vi "9217_UI.vi"(8 "error in (no error)":errorcluster, 11 "Node Ptr":T3 format="%.0x") -> (0 "error out":errorcluster)   [LabVIEW 2019, in "Modules.lvlib" / "9217.lvclass"]
uses:
  9217.lvclass
  <vilib>/NI VeriStand/Custom Device API/Custom Device Item Ref.ctl
  RSI Module/SubPanel Command.ctl
  _nicrio_cRIO-9217_SubPan_ConversionTime.ctl
  C:/Users/nitest/Desktop/Git 2019/niveristand-scan-engine-module-libraries/Source/RSI Module/RSI Module.lvclass
  9217.lvclass/9217.ctl
  RSI Module/RSI Module.lvclass
  <vilib>/NI VeriStand/Custom Device API/Custom Device API.lvlib
panel:
  in  "_9217 Config Data":T1={"Conversion Time"=0, "Degree Range"=[], "RTD_Type"=[1], "RTD_A"=[], "RTD_B"=[], "RTD_C"=[], "RTD_Ro"=[]} {"RTD_Type" items=["TCR3851"=1, "TCR3750"=2, "TCR3916"=3, "TCR3920"=4, "TCR3911"=5, "TCR3928"=6, "Custom"=0]; "Degree Range" items=["Raw Ohms", "Degrees Kelvin", "Degrees Celsius", "Degrees Fahrenheit", "Degrees Rankine"]; "Conversion Time" items=["200 ms", "2.5 ms"]}
  in  "_Measurement Units":u8(ring) items=["Raw Ohms", "Degrees Kelvin", "Degrees Celsius", "Degrees Fahrenheit", "Degrees Rankine"]
  in  "_RTD Type":u8(ring) items=["TCR3851"=1, "TCR3750"=2, "TCR3916"=3, "TCR3920"=4, "TCR3911"=5, "TCR3928"=6, "Custom"=0]
  out "Selected Channel Settings Label":string="Selected Channel Settings"
  out "RTD Coefficients Label":string="RTD Coefficients"
  in  "Ro":dbl
  in  "C":dbl
  in  "B":dbl
  in  "A":dbl
  in  "RTD Type":u8(ring) items=["TCR3851"=1, "TCR3750"=2, "TCR3916"=3, "TCR3920"=4, "TCR3911"=5, "TCR3928"=6, "Custom"=0]
  in  "Measurement Units":u8(ring) items=["Raw Ohms", "Degrees Kelvin", "Degrees Celsius", "Degrees Fahrenheit", "Degrees Rankine"]
  in  "Channels":i32[](listbox)=[0]
  in  "Conversion Time":T2 items=["200 ms", "2.5 ms"]
  in  "SubPanel Event":refnum<user-event>
  in  "Header":cluster{"Section Name":string}={"Section Name"="NI 9205 Settings"}
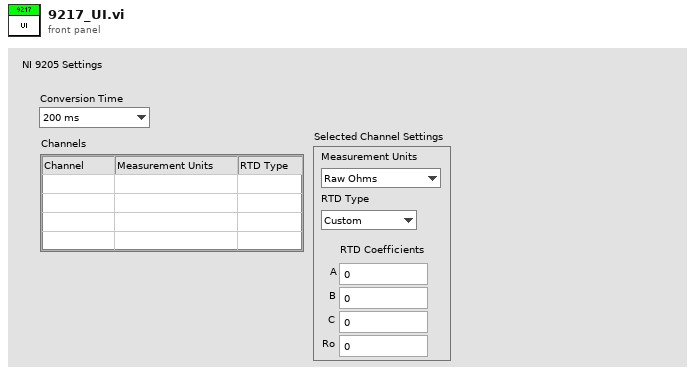
[diagram p1: front panel]
types:
  T1 = cluster{"Conversion Time":u16, "Degree Range":u8[], "RTD_Type":u8[], "RTD_A":dbl[], "RTD_B":dbl[], "RTD_C":dbl[], "RTD_Ro":dbl[]}
  T2 = typedef "Modules.lvlib/9217.lvclass/_nicrio_cRIO-9217_SubPan_ConversionTime.ctl" = u16
  T3 = typedef "Custom Device API.lvlib/Custom Device Item Ref.ctl" = u64
  T4 = typedef "LVStringsAndValuesArrayTypeDef_U8.ctl" = cluster{"String":string, "Value":u8}[]
  T5 = typedef "Modules.lvlib/RSI Module.lvclass/Module Models.ctl" = enum16{"Empty", "NI 9201", "NI 9203", "NI 9205", "NI 9206", "NI 9207", "NI 9208", "NI 9209", "NI 9210", "NI 9211", "NI 9212", "NI 9213", "NI 9214", "NI 9215", "NI 9216", "NI 9217", "NI 9219", "NI 9220", "NI 9221", "NI 9222", "NI 9223", "NI 9224", "NI 9225", "NI 9226", "NI 9227", "NI 9228", "NI 9229", "NI 9233", "NI 9234", "NI 9235", "NI 9236", "NI 9237", "NI 9239", "NI 9242", "NI 9244", "NI 9253", "NI 9263", "NI 9264", "NI 9265", "NI 9266", "NI 9269", "NI 9344", "NI 9350", "NI 9375", "NI 9401", "NI 9402", "NI 9403", "NI 9411", "NI 9421", "NI 9422", "NI 9423", "NI 9425", "NI 9426", "NI 9435", "NI 9436", "NI 9437", "NI 9472", "NI 9474", "NI 9475", "NI 9476", "NI 9477", "NI 9478", "NI 9481", "NI 9482", "NI 9485"}
  T6 = cluster{"Ohm degree range":u32, "RTD type":u32, "RTD user-defined A constant":dbl, "RTD user-defined B constant":dbl, "RTD user-defined C constant":dbl, "RTD user-defined Ro constant":dbl}[]
  T7 = typedef "Modules.lvlib/RSI Module.lvclass/SubPanel Command.ctl" = enum16{"Stop"}
  T8 = typedef "Custom Device API.lvlib/Custom Device Channel.ctl" = cluster{"Type":T9, "Units":string, "Default Value":dbl, "Faultable":bool, "Scalable":bool}
  T9 = typedef "Custom Device API.lvlib/Custom Device Channel Type.ctl" = enum16{"Input", "Output"}
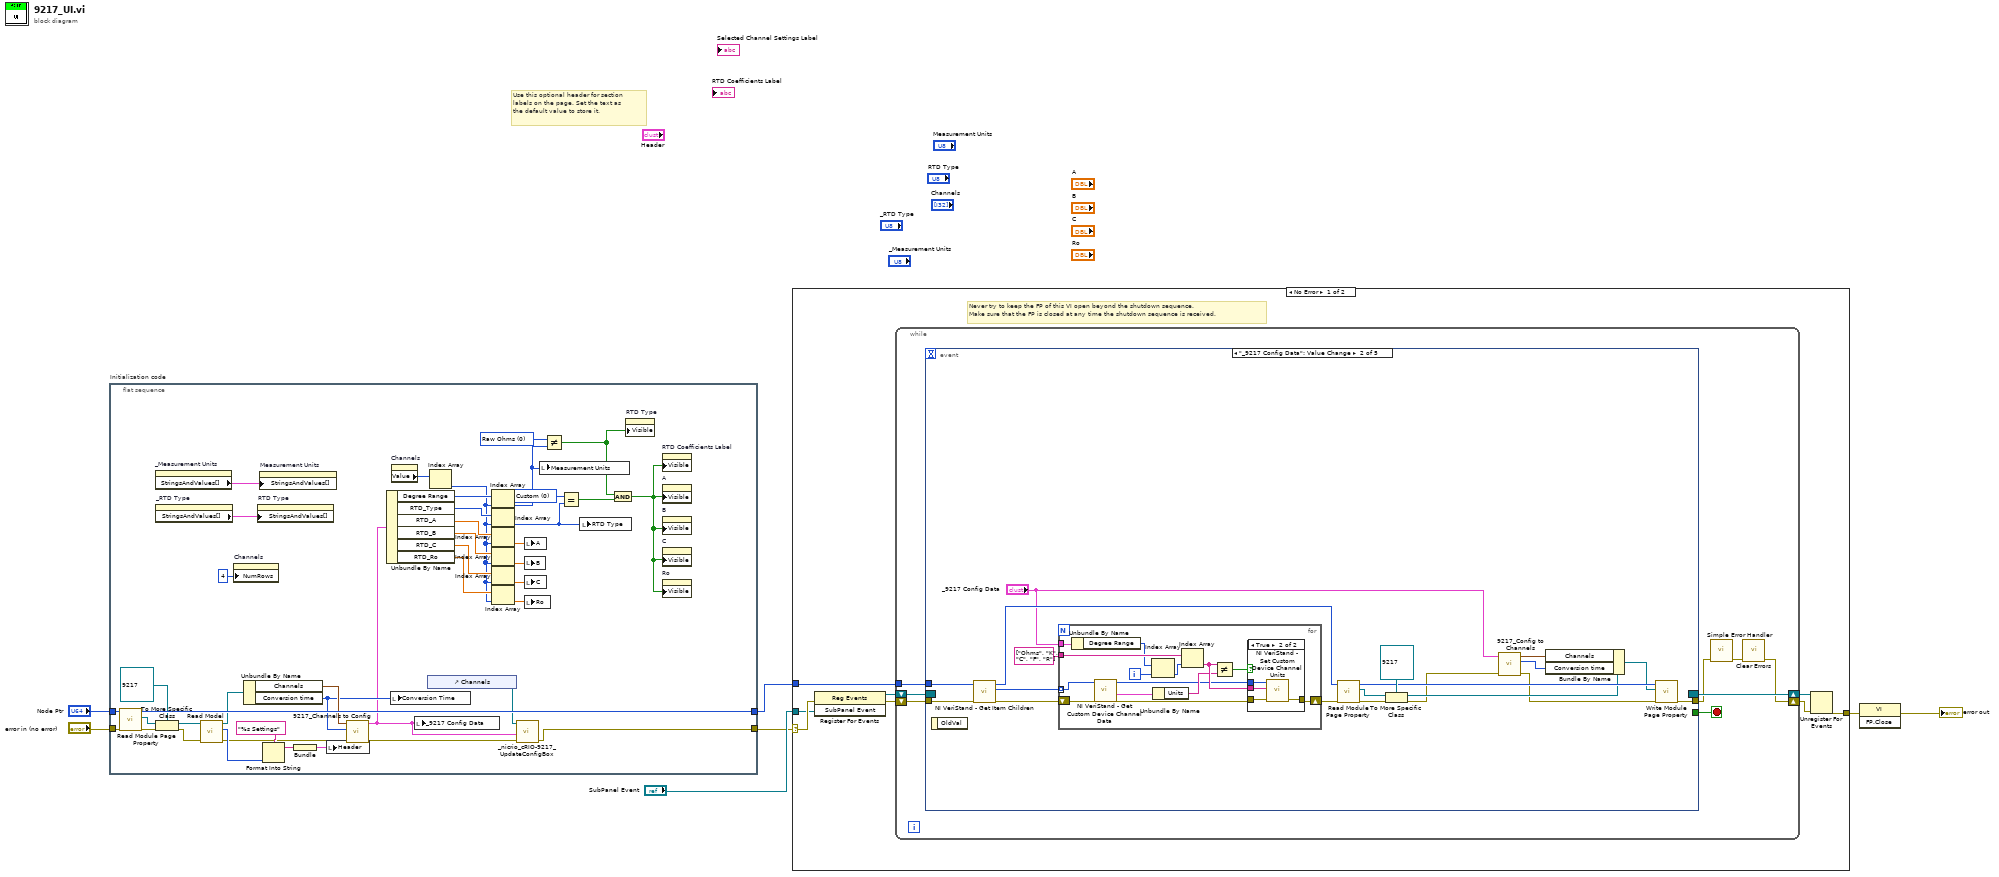
[diagram p0: block diagram]
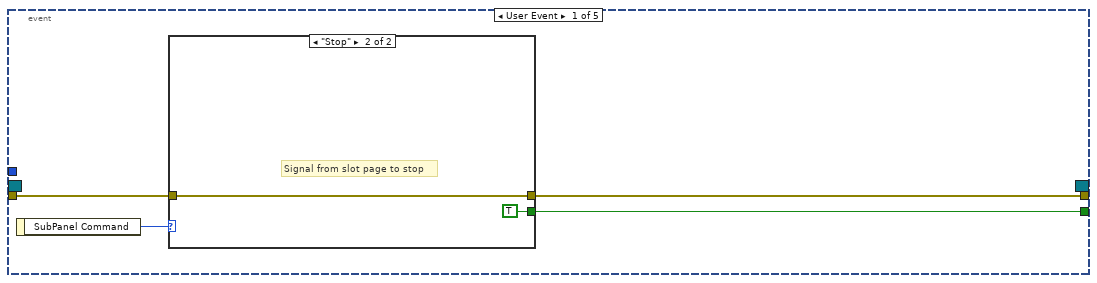
[diagram p2: hidden frame]
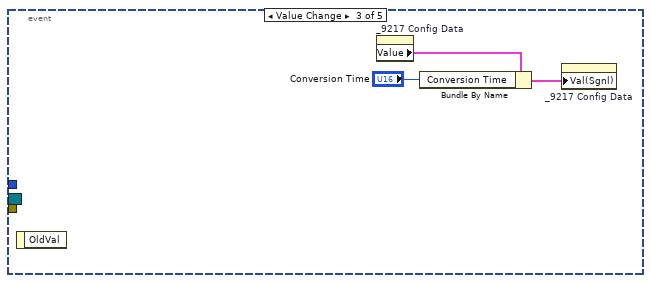
[diagram p5: hidden frame]
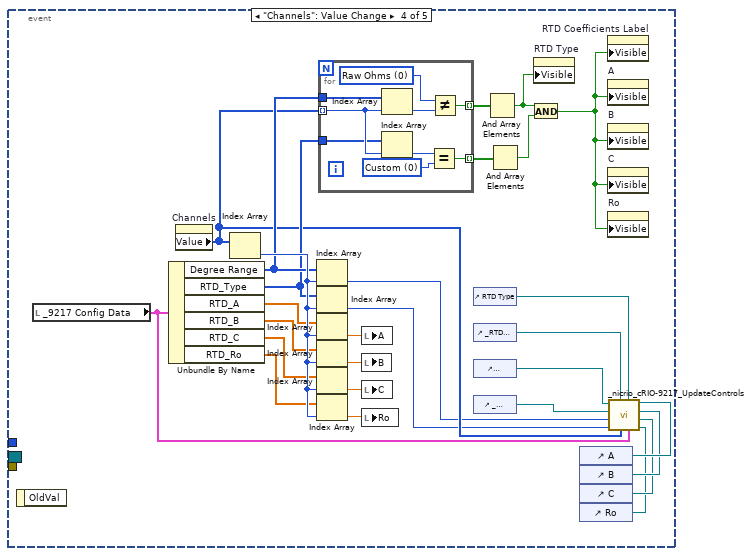
[diagram p6: hidden frame]
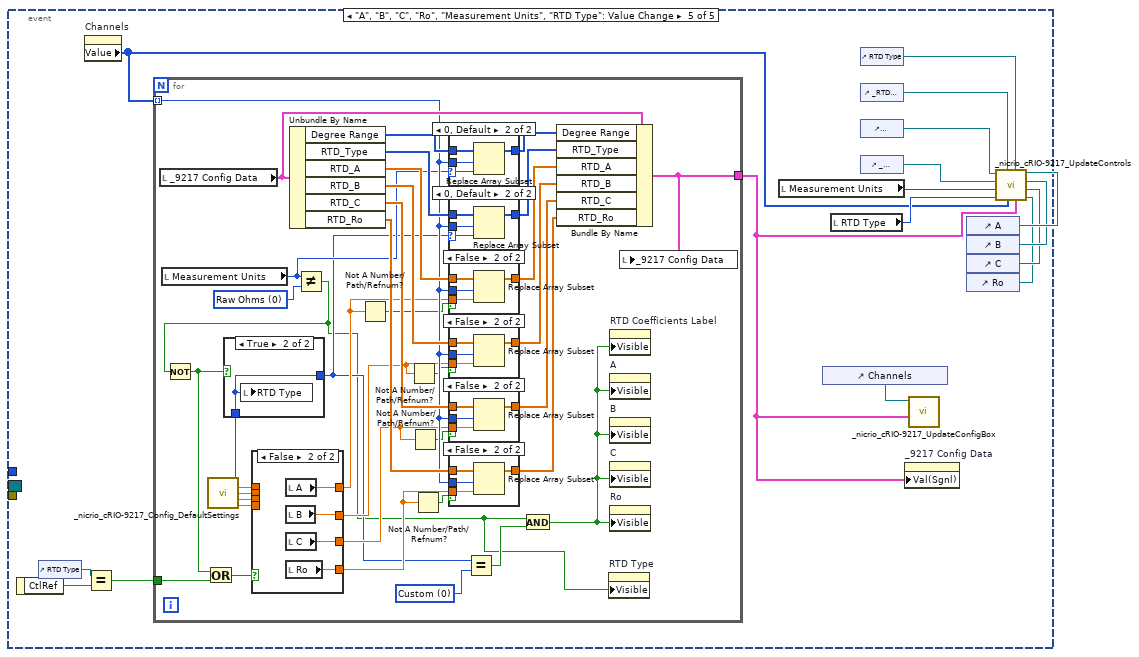
[diagram p7: hidden frame]
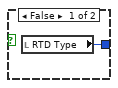
[diagram p8: hidden frame]
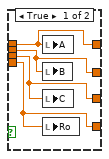
[diagram p9: hidden frame]
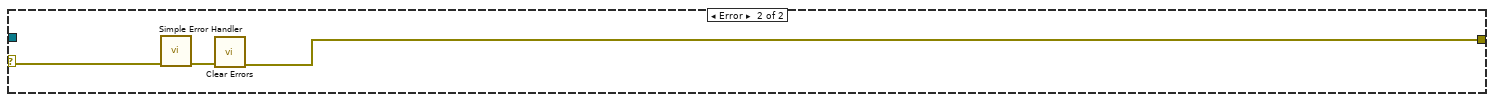
[diagram p16: hidden frame]
diagram:
  # "Use this optional header for section labels on the page. Set the text as the default value to store it."
  n1 = flat-sequence "Initialization code" {
    tunnel: "error in (no error)" -> [w48]
    tunnel: "Node Ptr" -> [w49]
    tunnel: [w31] -> w1
    tunnel: [w47] -> w4
    frame #0 {
      w15 = u8 0 items=["Raw Ohms", "Degrees Kelvin", "Degrees Celsius", "Degrees Fahrenheit", "Degrees Rankine"] ("Measurement Units")
      w16 = u8 0 items=["TCR3851"=1, "TCR3750"=2, "TCR3916"=3, "TCR3920"=4, "TCR3911"=5, "TCR3928"=6, "Custom"=0] ("RTD Type")
      n2 = call "Read Module Page Property.vi"("error in (no error)"=w48, "Node Ptr In"=w49) -> ("error out"=w46:errorcluster, "RSI Module"=w44:refnum<class "RSI Module.lvclass">, "Node Ptr Out"=w47:T3)  [unwired: 7 in]
      n3 = property on="_Measurement Units" class="Ring (strict)"() -> ("StringsAndValues[]"=w10:T4)  [unwired: 2 in, 2 out]
      n4 = property on="_RTD Type" class="Ring (strict)"() -> ("StringsAndValues[]"=w9:T4)  [unwired: 2 in, 2 out]
      n5 = To More Specific Class(target class=refnum<class "9217.lvclass"> refnum ("9205 in"), reference=w44, error in=w46) -> (specific class reference=w43:refnum<class "9217.lvclass">, error out=w42:errorcluster)
      n6 = call "Read Model.vi"("error in (no error)"=w42, "RSI Module in"=w43) -> ("error out"=w34:errorcluster, "Model"=w40:T5, "RSI Module out"=w37:refnum<class "9217.lvclass">)  [unwired: 7 in]
      n7 = property on="Channels" class="MCListbox (strict)"("NumRows"=u32 4 ("Number of Rows")) -> ()  [unwired: 2 in, 2 out]
      n8 = Unbundle By Name(w37) -> ("Channels"=w36:T6, "Conversion time"=w35:u32)
      n9 = property on="RTD Type" class="Ring (strict)"("StringsAndValues[]"=w9) -> ()  [unwired: 2 in, 2 out]
      n10 = property on="Measurement Units" class="Ring (strict)"("StringsAndValues[]"=w10) -> ()  [unwired: 2 in, 2 out]
      n11 = Format Into String(format string="%s Settings", w40) -> (resulting string=w38:string)  [unwired: 2 in, 1 out]
      n12 = Bundle(w38) -> (w41:cluster{string})  [unwired: 1 in]
      n13 = local write "Header"(w41) -> ()
      n14 = call "9217_Channels to Config.vi"("error in (no error)"=w34, "Conversion Time"=w35, "Channels"=w36) -> ("error out"=w32:errorcluster, "_9217 Config Data"=w30:T1)  [unwired: 7 in]
      n15 = Unbundle By Name(w30) -> ("Degree Range"=w28:u8[], "RTD_Type"=w27:u8[], "RTD_A"=w26:dbl[], "RTD_B"=w25:dbl[], "RTD_C"=w24:dbl[], "RTD_Ro"=w23:dbl[])
      n16 = local write "Conversion Time"(w35) -> ()
      n17 = property on="Channels" class="MCListbox (strict)"() -> ("Value"=w29:i32[])  [unwired: 2 in, 2 out]
      n18 = local write "_9217 Config Data"(w30) -> ()
      n19 = control-ref of="Channels"() -> (w33:refnum<vi>)
      n20 = Index Array(array=w29) -> (element=w22:i32)  [unwired: 1 in]
      n21 = Index Array(array=w28, index=w22) -> (element=w14:u8)
      n22 = Index Array(array=w27, index=w22) -> (element=w17:u8)
      n23 = Index Array(array=w26, index=w22) -> (element=w18:dbl)
      n24 = Index Array(array=w25, index=w22) -> (element=w19:dbl)
      n25 = Index Array(array=w24, index=w22) -> (element=w20:dbl)
      n26 = Index Array(array=w23, index=w22) -> (element=w21:dbl)
      n27 = call "_nicrio_cRIO-9217_UpdateConfigBox.vi"("error in (no error)"=w32, "_9217 Config"=w30, "_Channel Refnum"=w33) -> ("error out"=w31:errorcluster)  [unwired: 8 in]
      n28 = local write "A"(w18) -> ()
      n29 = local write "B"(w19) -> ()
      n30 = local write "C"(w20) -> ()
      n31 = local write "Ro"(w21) -> ()
      n32 = local write "Measurement Units"(w14) -> ()
      n33 = Not Equal?(x=w15, y=w14) -> (x != y?=w12:bool)
      n34 = Equal?(x=w16, y=w17) -> (x = y?=w13:bool)
      n35 = local write "RTD Type"(w17) -> ()
      n36 = And(x=w12, y=w13) -> (x .and. y?=w11:bool)
      n37 = property on="RTD Type" class="Ring (strict)"("Visible"=w12) -> ()  [unwired: 2 in, 2 out]
      n38 = property on="RTD Coefficients Label" class="Str"("Visible"=w11) -> ()  [unwired: 2 in, 2 out]
      n39 = property on="A" class="DigNum (strict)"("Visible"=w11) -> ()  [unwired: 2 in, 2 out]
      n40 = property on="B" class="DigNum (strict)"("Visible"=w11) -> ()  [unwired: 2 in, 2 out]
      n41 = property on="C" class="DigNum (strict)"("Visible"=w11) -> ()  [unwired: 2 in, 2 out]
      n42 = property on="Ro" class="DigNum (strict)"("Visible"=w11) -> ()  [unwired: 2 in, 2 out]
    }
  }
  n43 = case shown="No Error" w1 {
    selector: w1 -> [w51 w247]
    tunnel: [w55 w245] -> w7
    tunnel: w4 -> [w52 _]
    tunnel: "SubPanel Event" -> [w50 _]
    frame No Error {
      # "Never try to keep the FP of this VI open beyond the shutdown sequence.\nMake sure that the FP is closed at any time the shutdown sequence is received."
      n44 = register-events(error in=w51, w50) -> (reference out=w53:refnum<event-registration>, error out=w54:errorcluster)  [unwired: 1 in]
      n45 = while {
        tunnel: w52 -> [w61]
        shift-right: [w58] -> w56
        shift-left: w54 -> [w64]
        shift-right: [w65] -> w57
        shift-left: w53 -> [w63]
        stop <- w62 stop-if-true
        n46 = event shown="[1] \"_9217 Config Data\": Value Change" {
          selector: w63 -> [_ _ _ _ _]
          dyn-events: [_ _ _ _ _] -> w65
          timeout: _ -> [_ _ _ _ _]
          tunnel: w64 -> [w68 w79 _ _ _]
          tunnel: [w67 _ _ _ _] -> w62
          tunnel: [w66 w87 _ _ _] -> w60
          tunnel: w61 -> [_ w80 _ _ _]
          event User Event {
            n47 = event-data() -> ("SubPanel Command"=w69:T7)  [unwired: 1 out]
            n48 = case shown="\"Stop\"" w69 {
              tunnel: w68 -> [w70 w71]
              tunnel: [w70 w71] -> w66
              tunnel: [_ TRUE] -> w67
              frame Default {
              }
              frame "Stop" {
                # "Signal from slot page to stop"
              }
            }
          }
          event "_9217 Config Data": Value Change {
            n49 = event-data() -> ()  [unwired: 2 out]
            n50 = call <vilib>:"NI VeriStand - Get Item Children.vi"("error in (no error)"=w79, "Item Ref in"=w80) -> ("error out"=w78:errorcluster, "Child Refs"=w77:T3[], "Item Ref out"=w76:T3)  [unwired: 6 in, 1 out]
            n51 = for {
              tunnel: w77 -> [w96] mode=indexing
              shift-right: [w97] -> w75
              shift-left: w78 -> [w99]
              tunnel: "_9217 Config Data" -> [w105]
              tunnel: string[] ["Ohms", "K", "C", "F", "R"] -> [w104]
              i -> [w93]
              n52 = Unbundle By Name(w105) -> ("Degree Range"=w94:u8[])
              n53 = call <vilib>:"NI VeriStand - Get Custom Device Channel Data.vi"("error in (no error)"=w99, "Channel Ref in"=w96) -> ("error out"=w98:errorcluster, "Channel"=w101:T8, "Channel Ref out"=w95:T3)  [unwired: 4 in, 3 out]
              n54 = Index Array(array=w94, index=w93) -> (element=w92:u8)
              n55 = Unbundle By Name(w101) -> ("Units"=w100:string)
              n56 = Index Array(array=w104, index=w92) -> (element=w102:string)
              n57 = Not Equal?(x=w102, y=w100) -> (x != y?=w103:bool)
              n58 = case shown="True" w103 {
                tunnel: w95 -> [_ w110]
                tunnel: w102 -> [_ w109]
                tunnel: w98 -> [w106 w108]
                tunnel: [w106 w107] -> w97
                frame False {
                }
                frame True {
                  n59 = call <vilib>:"NI VeriStand - Set Custom Device Channel Units.vi"("error in (no error)"=w108, "Units"=w109, "Channel Ref in"=w110) -> ("error out"=w107:errorcluster)  [unwired: 7 in, 1 out]
                }
              }
            }
            n60 = call "Read Module Page Property.vi"("error in (no error)"=w75, "Node Ptr In"=w76) -> ("error out"=w89:errorcluster, "RSI Module"=w90:refnum<class "RSI Module.lvclass">, "Node Ptr Out"=w88:T3)  [unwired: 7 in]
            n61 = To More Specific Class(target class=refnum<class "9217.lvclass"> refnum ("9205 in"), reference=w90, error in=w89) -> (specific class reference=w86:refnum<class "9217.lvclass">, error out=w83:errorcluster)
            n62 = call "9217_Config to Channels.vi"("error in (no error)"=w83, "_9217 Config Data"="_9217 Config Data") -> ("error out"=w82:errorcluster, "Conversion Time"=w81:u16, "Channels"=w84:T6)  [unwired: 7 in]
            n63 = Bundle By Name(cluster=w86, "Channels"=w84, "Conversion time"=w81) -> (w85:refnum<class "9217.lvclass">)
            n64 = call "Write Module Page Property.vi"("error in (no error)"=w82, "RSI Module"=w85, "Node Ptr In"=w88) -> ("error out"=w87:errorcluster)  [unwired: 6 in, 2 out]
          }
          event Value Change {
            n65 = event-data() -> ()  [unwired: 2 out]
            n66 = property on="_9217 Config Data" class="Clust (strict)"() -> ("Value"=w113:T1)  [unwired: 2 in, 2 out]
            n67 = Bundle By Name(cluster=w113, "Conversion Time"="Conversion Time") -> (w111:T1)
            n68 = property on="_9217 Config Data" class="Clust (strict)"("Val(Sgnl)"=w111) -> ()  [unwired: 2 in, 2 out]
          }
          event "Channels": Value Change {
            n69 = event-data() -> ()  [unwired: 2 out]
            n70 = local read "_9217 Config Data"() -> (w121:T1)
            n71 = Unbundle By Name(w121) -> ("Degree Range"=w132:u8[], "RTD_Type"=w131:u8[], "RTD_A"=w133:dbl[], "RTD_B"=w134:dbl[], "RTD_C"=w135:dbl[], "RTD_Ro"=w136:dbl[])
            n72 = property on="Channels" class="MCListbox (strict)"() -> ("Value"=w120:i32[])  [unwired: 2 in, 2 out]
            n73 = Index Array(array=w120) -> (element=w137:i32)  [unwired: 1 in]
            n74 = Index Array(array=w132, index=w137) -> (element=w118:u8)
            n75 = Index Array(array=w131, index=w137) -> (element=w119:u8)
            n76 = Index Array(array=w133, index=w137) -> (element=w141:dbl)
            n77 = Index Array(array=w134, index=w137) -> (element=w140:dbl)
            n78 = Index Array(array=w135, index=w137) -> (element=w139:dbl)
            n79 = Index Array(array=w136, index=w137) -> (element=w138:dbl)
            n80 = for {
              tunnel: w120 -> [w150] mode=indexing
              tunnel: w132 -> [w149]
              tunnel: w131 -> [w148]
              tunnel: [w143] -> w130 mode=indexing
              tunnel: [w142] -> w129 mode=indexing
              w144 = u8 0 items=["TCR3851"=1, "TCR3750"=2, "TCR3916"=3, "TCR3920"=4, "TCR3911"=5, "TCR3928"=6, "Custom"=0] ("RTD Type")
              w147 = u8 0 items=["Raw Ohms", "Degrees Kelvin", "Degrees Celsius", "Degrees Fahrenheit", "Degrees Rankine"] ("Measurement Units")
              n81 = Index Array(array=w149, index=w150) -> (element=w146:u8)
              n82 = Index Array(array=w148, index=w150) -> (element=w145:u8)
              n83 = Equal?(x=w145, y=w144) -> (x = y?=w142:bool)
              n84 = Not Equal?(x=w147, y=w146) -> (x != y?=w143:bool)
            }
            n85 = local write "A"(w141) -> ()
            n86 = local write "B"(w140) -> ()
            n87 = local write "C"(w139) -> ()
            n88 = local write "Ro"(w138) -> ()
            n89 = control-ref of="RTD Type"() -> (w114:refnum<vi>)
            n90 = control-ref of="_RTD Type"() -> (w115:refnum<vi>)
            n91 = control-ref of="Measurement Units"() -> (w116:refnum<vi>)
            n92 = control-ref of="_Measurement Units"() -> (w117:refnum<vi>)
            n93 = And Array Elements(Boolean array=w130) -> (logical AND=w127:bool)
            n94 = And Array Elements(Boolean array=w129) -> (logical AND=w128:bool)
            n95 = And(x=w127, y=w128) -> (x .and. y?=w126:bool)
            n96 = property on="RTD Type" class="Ring (strict)"("Visible"=w127) -> ()  [unwired: 2 in, 2 out]
            n97 = control-ref of="A"() -> (w125:refnum<vi>)
            n98 = control-ref of="B"() -> (w124:refnum<vi>)
            n99 = control-ref of="C"() -> (w123:refnum<vi>)
            n100 = control-ref of="Ro"() -> (w122:refnum<vi>)
            n101 = property on="RTD Coefficients Label" class="Str"("Visible"=w126) -> ()  [unwired: 2 in, 2 out]
            n102 = property on="A" class="DigNum (strict)"("Visible"=w126) -> ()  [unwired: 2 in, 2 out]
            n103 = property on="B" class="DigNum (strict)"("Visible"=w126) -> ()  [unwired: 2 in, 2 out]
            n104 = property on="C" class="DigNum (strict)"("Visible"=w126) -> ()  [unwired: 2 in, 2 out]
            n105 = property on="Ro" class="DigNum (strict)"("Visible"=w126) -> ()  [unwired: 2 in, 2 out]
            n106 = call "_nicrio_cRIO-9217_UpdateControls.vi"("D"=w122, "C"=w123, "B"=w124, "A"=w125, "9217 Config"=w121, "TypeControl"=w114, "Values"=w120, "TypeTypeDef"=w115, "RTD Type"=w119, "Units"=w118, "UnitsControl"=w117, "UnitsTypeDef"=w116) -> ()
          }
          event "A", "B", "C", "Ro", "Measurement Units", "RTD Type": Value Change {
            n107 = event-data() -> ("CtlRef"=w155:refnum<vi>)  [unwired: 1 out]
            n108 = control-ref of="RTD Type"() -> (w154:refnum<vi>)
            n109 = property on="Channels" class="MCListbox (strict)"() -> ("Value"=w156:i32[])  [unwired: 2 in, 2 out]
            n110 = Equal?(x=w154, y=w155) -> (x = y?=w153:bool)
            n111 = for {
              tunnel: w156 -> [w183] mode=indexing
              tunnel: [w203] -> w151
              tunnel: w153 -> [w189]
              w170 = u8 0 items=["TCR3851"=1, "TCR3750"=2, "TCR3916"=3, "TCR3920"=4, "TCR3911"=5, "TCR3928"=6, "Custom"=0] ("RTD Type")
              w190 = u8 0 items=["Raw Ohms", "Degrees Kelvin", "Degrees Celsius", "Degrees Fahrenheit", "Degrees Rankine"] ("Measurement Units")
              n112 = local read "_9217 Config Data"() -> (w204:T1)
              n113 = local read "Measurement Units"() -> (w174:u8)
              n114 = call "_nicrio_cRIO-9217_Config_DefaultSettings.vi"() -> ("RTD Types"=w172:u8, "RTD_A"=w187:dbl, "RTD_B"=w186:dbl, "RTD_C"=w185:dbl, "RTD_Ro"=w184:dbl)  [unwired: 9 in, 2 out]
              n115 = Unbundle By Name(w204) -> ("Degree Range"=w202:u8[], "RTD_Type"=w200:u8[], "RTD_A"=w198:dbl[], "RTD_B"=w197:dbl[], "RTD_C"=w196:dbl[], "RTD_Ro"=w195:dbl[])
              n116 = Not Equal?(x=w174, y=w190) -> (x != y?=w167:bool)
              n117 = Not(x=w167) -> (.not. x?=w173:bool)
              n118 = Or(x=w173, y=w189) -> (x .or. y?=w188:bool)
              n119 = case shown="True" w173 {
                tunnel: [w205 w206] -> w171
                tunnel: w172 -> [_ w206]
                frame False {
                  n120 = local read "RTD Type"() -> (w205:u8)
                }
                frame True {
                  n121 = local write "RTD Type"(w206) -> ()
                }
              }
              n122 = case shown="False" w188 {
                tunnel: w187 -> [w210 _]
                tunnel: w186 -> [w209 _]
                tunnel: w185 -> [w208 _]
                tunnel: w184 -> [w207 _]
                tunnel: [w210 w214] -> w176
                tunnel: [w209 w213] -> w177
                tunnel: [w208 w212] -> w179
                tunnel: [w207 w211] -> w181
                frame True {
                  n123 = local write "A"(w210) -> ()
                  n124 = local write "B"(w209) -> ()
                  n125 = local write "C"(w208) -> ()
                  n126 = local write "Ro"(w207) -> ()
                }
                frame False {
                  n127 = local read "A"() -> (w214:dbl)
                  n128 = local read "B"() -> (w213:dbl)
                  n129 = local read "C"() -> (w212:dbl)
                  n130 = local read "Ro"() -> (w211:dbl)
                }
              }
              n131 = Not A Number/Path/Refnum?(number/path/refnum=w176) -> (NaN/Path/Refnum?=w175:bool)
              n132 = Not A Number/Path/Refnum?(number/path/refnum=w177) -> (NaN/Path/Refnum?=w178:bool)
              n133 = Not A Number/Path/Refnum?(number/path/refnum=w179) -> (NaN/Path/Refnum?=w180:bool)
              n134 = Not A Number/Path/Refnum?(number/path/refnum=w181) -> (NaN/Path/Refnum?=w182:bool)
              n135 = case shown="0, Default" w174 {
                selector: w174 -> [_ w243]
                tunnel: [w240 w244] -> w201
                tunnel: w202 -> [w240 w242]
                tunnel: w183 -> [_ w241]
                frame 99 {
                }
                frame 0, Default {
                  n136 = Replace Array Subset(array=w242, new element=w243, index=w241) -> (w244:u8[])
                }
              }
              n137 = case shown="0, Default" w171 {
                selector: w171 -> [_ w238]
                tunnel: [w235 w239] -> w199
                tunnel: w200 -> [w235 w237]
                tunnel: w183 -> [_ w236]
                frame 99 {
                }
                frame 0, Default {
                  n138 = Replace Array Subset(array=w237, new element=w238, index=w236) -> (w239:u8[])
                }
              }
              n139 = case shown="False" w175 {
                tunnel: [w230 w234] -> w194
                tunnel: w198 -> [w230 w233]
                tunnel: w183 -> [_ w232]
                tunnel: w176 -> [_ w231]
                frame True {
                }
                frame False {
                  n140 = Replace Array Subset(array=w233, new element=w231, index=w232) -> (w234:dbl[])
                }
              }
              n141 = case shown="False" w178 {
                tunnel: [w225 w229] -> w193
                tunnel: w197 -> [w225 w228]
                tunnel: w183 -> [_ w227]
                tunnel: w177 -> [_ w226]
                frame True {
                }
                frame False {
                  n142 = Replace Array Subset(array=w228, new element=w226, index=w227) -> (w229:dbl[])
                }
              }
              n143 = case shown="False" w180 {
                tunnel: [w220 w224] -> w192
                tunnel: w196 -> [w220 w223]
                tunnel: w183 -> [_ w222]
                tunnel: w179 -> [_ w221]
                frame True {
                }
                frame False {
                  n144 = Replace Array Subset(array=w223, new element=w221, index=w222) -> (w224:dbl[])
                }
              }
              n145 = case shown="False" w182 {
                tunnel: [w215 w219] -> w191
                tunnel: w195 -> [w215 w218]
                tunnel: w183 -> [_ w217]
                tunnel: w181 -> [_ w216]
                frame True {
                }
                frame False {
                  n146 = Replace Array Subset(array=w218, new element=w216, index=w217) -> (w219:dbl[])
                }
              }
              n147 = Equal?(x=w171, y=w170) -> (x = y?=w168:bool)
              n148 = And(x=w167, y=w168) -> (x .and. y?=w169:bool)
              n149 = Bundle By Name(cluster=w204, "Degree Range"=w201, "RTD_Type"=w199, "RTD_A"=w194, "RTD_B"=w193, "RTD_C"=w192, "RTD_Ro"=w191) -> (w203:T1)
              n150 = property on="RTD Type" class="Ring (strict)"("Visible"=w167) -> ()  [unwired: 2 in, 2 out]
              n151 = property on="RTD Coefficients Label" class="Str"("Visible"=w169) -> ()  [unwired: 2 in, 2 out]
              n152 = property on="A" class="DigNum (strict)"("Visible"=w169) -> ()  [unwired: 2 in, 2 out]
              n153 = property on="B" class="DigNum (strict)"("Visible"=w169) -> ()  [unwired: 2 in, 2 out]
              n154 = property on="C" class="DigNum (strict)"("Visible"=w169) -> ()  [unwired: 2 in, 2 out]
              n155 = property on="Ro" class="DigNum (strict)"("Visible"=w169) -> ()  [unwired: 2 in, 2 out]
              n156 = local write "_9217 Config Data"(w203) -> ()
            }
            n157 = local read "Measurement Units"() -> (w158:u8)
            n158 = control-ref of="Channels"() -> (w152:refnum<vi>)
            n159 = local read "RTD Type"() -> (w157:u8)
            n160 = control-ref of="RTD Type"() -> (w159:refnum<vi>)
            n161 = control-ref of="_RTD Type"() -> (w160:refnum<vi>)
            n162 = control-ref of="Measurement Units"() -> (w161:refnum<vi>)
            n163 = control-ref of="_Measurement Units"() -> (w162:refnum<vi>)
            n164 = property on="_9217 Config Data" class="Clust (strict)"("Val(Sgnl)"=w151) -> ()  [unwired: 2 in, 2 out]
            n165 = call "_nicrio_cRIO-9217_UpdateConfigBox.vi"("_9217 Config"=w151, "_Channel Refnum"=w152) -> ()  [unwired: 9 in, 1 out]
            n166 = control-ref of="A"() -> (w166:refnum<vi>)
            n167 = control-ref of="B"() -> (w165:refnum<vi>)
            n168 = control-ref of="C"() -> (w164:refnum<vi>)
            n169 = control-ref of="Ro"() -> (w163:refnum<vi>)
            n170 = call "_nicrio_cRIO-9217_UpdateControls.vi"("D"=w163, "C"=w164, "B"=w165, "A"=w166, "9217 Config"=w151, "TypeControl"=w159, "Values"=w156, "TypeTypeDef"=w160, "RTD Type"=w157, "Units"=w158, "UnitsControl"=w162, "UnitsTypeDef"=w161) -> ()
          }
        }
        n171 = call <vilib>:"Simple Error Handler.vi"("error in (no error)"=w60) -> ("error out"=w59:errorcluster)  [unwired: 1 in, 7 out]
        n172 = call <vilib>:"Clear Errors.vi"("error in (no error)"=w59) -> ("error out"=w58:errorcluster)  [unwired: 1 in, 5 out]
      }
      n173 = Unregister For Events(event registration refnum=w57, error in=w56) -> (error out=w55:errorcluster)
    }
    frame Error {
      n174 = call <vilib>:"Simple Error Handler.vi"("error in (no error)"=w247) -> ("error out"=w246:errorcluster)  [unwired: 1 in, 7 out]
      n175 = call <vilib>:"Clear Errors.vi"("error in (no error)"=w246) -> ("error out"=w245:errorcluster)  [unwired: 1 in, 5 out]
    }
  }
  n176 = invoke class="VI" method="FP.Close"(error in=w7) -> (error out=→"error out":errorcluster)  [unwired: 2 in, 2 out]
